vi "FGV_tristate_indicator_OBJ_test.vi"(6 "boolean_indicator_refnum":refnum<vi>, 7 "options":T1, 8 "error_in":errorcluster) -> (0 "error_out":errorcluster)   [LabVIEW 2019]
uses:
  FGV_tristate_indicator_OBJ_test.ctl
  _misc/AULocalize/SubVIs/Get Localized Phrase Compact Interface 1D.vi
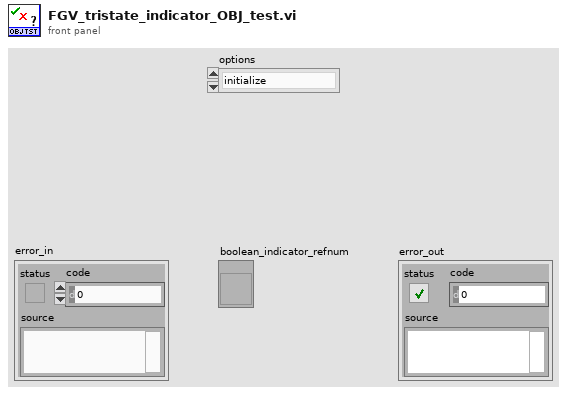
[diagram p1: front panel]
types:
  T1 = typedef "FGV_tristate_indicator_OBJ_test.ctl" = enum16{"initialize", "ready", "pending", "OK", "NOK", "part_NOK", "routing_NOK", "repeat_NOK", "timeout", "translate", "error"}
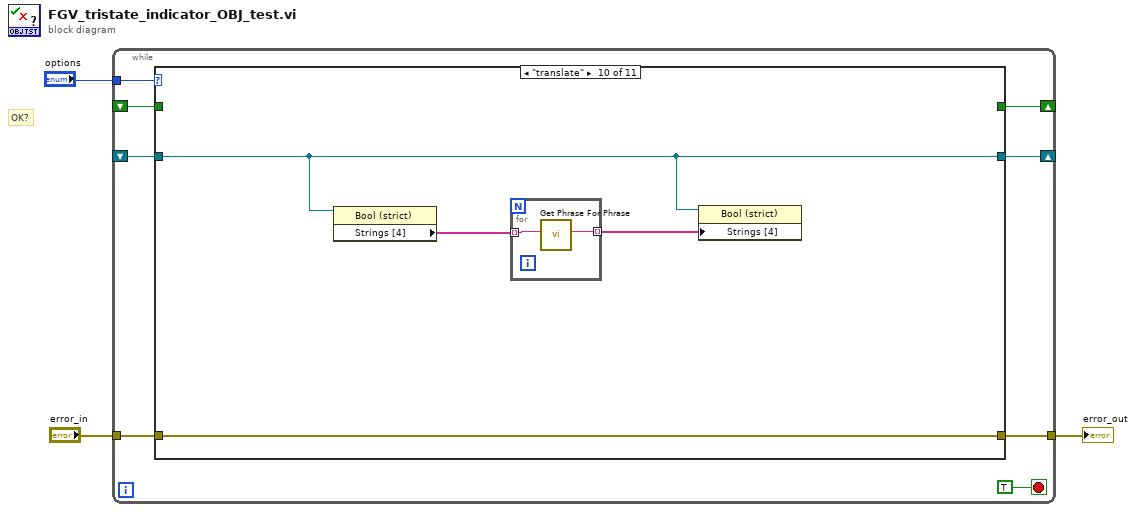
[diagram p0: block diagram]
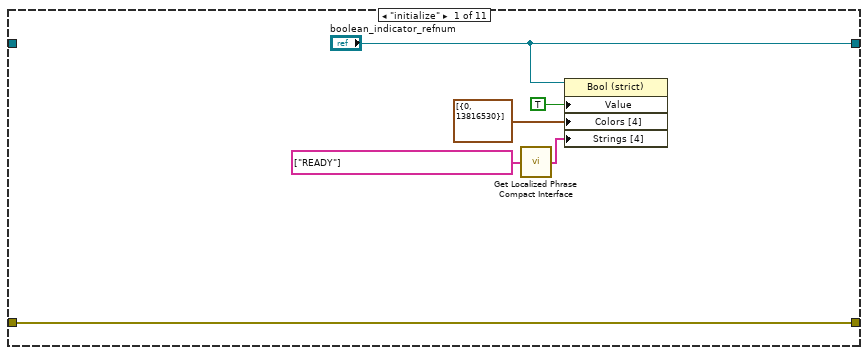
[diagram p2: hidden frame]
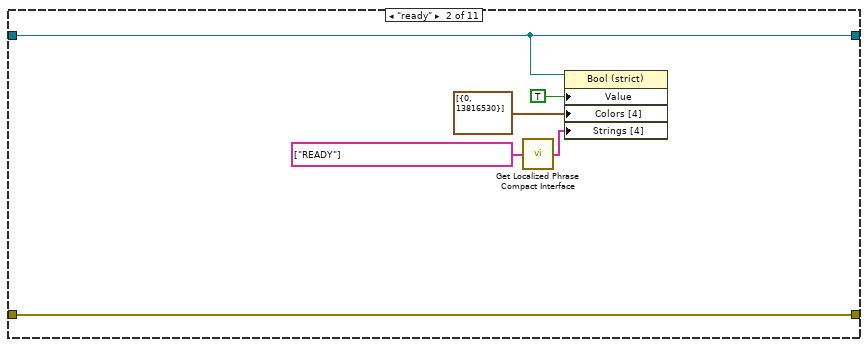
[diagram p3: hidden frame]
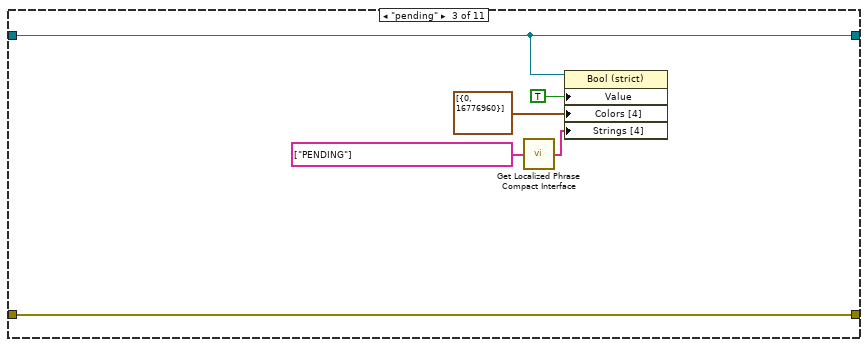
[diagram p4: hidden frame]
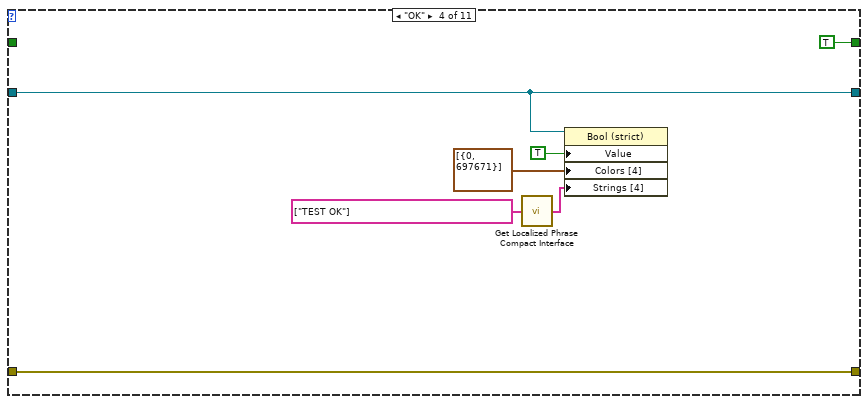
[diagram p5: hidden frame]
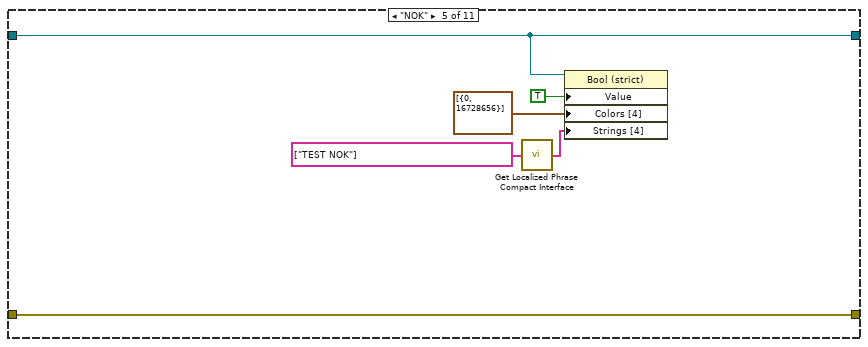
[diagram p6: hidden frame]
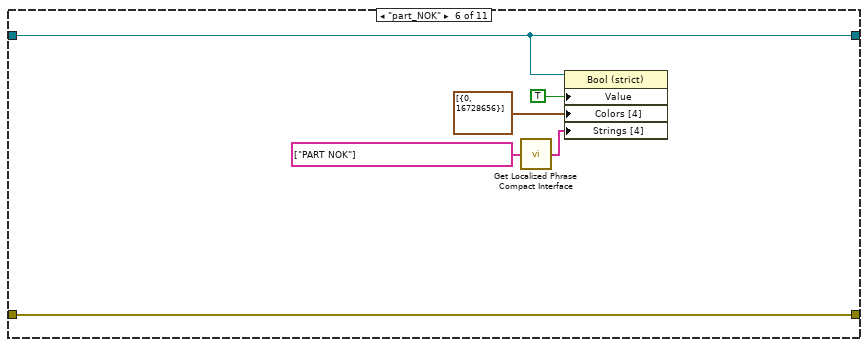
[diagram p7: hidden frame]
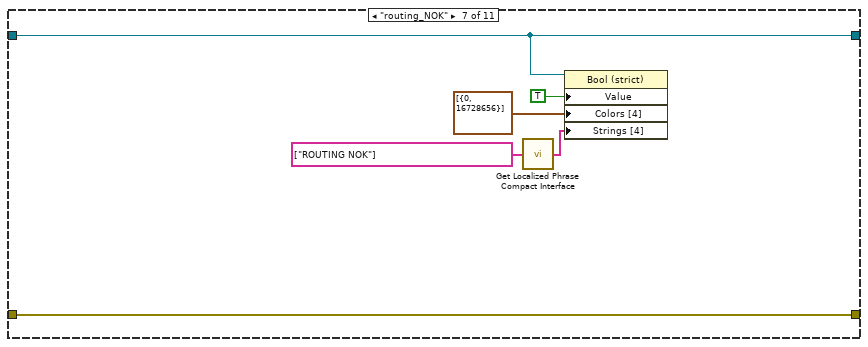
[diagram p8: hidden frame]
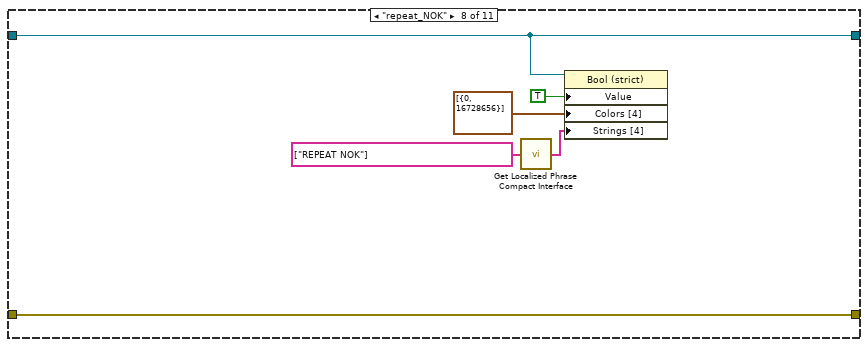
[diagram p9: hidden frame]
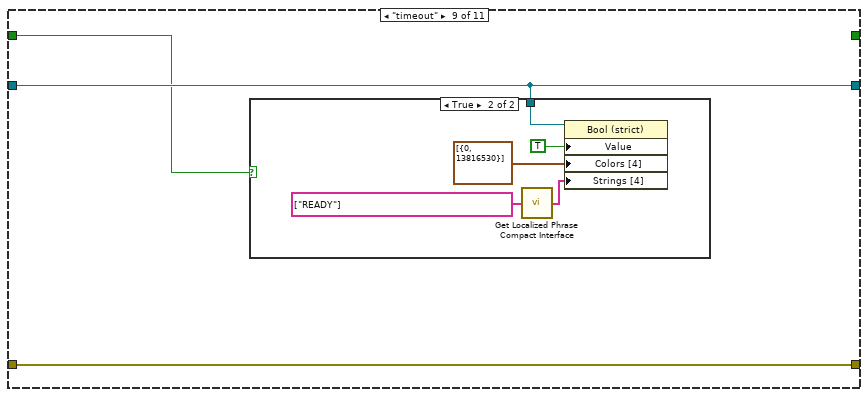
[diagram p10: hidden frame]
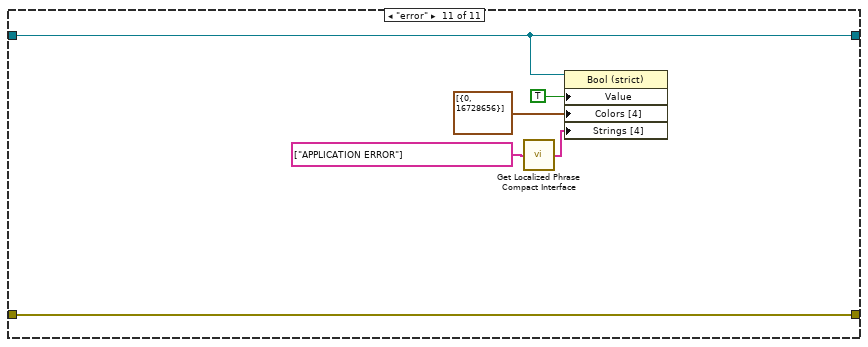
[diagram p12: hidden frame]
diagram:
  # "OK?"
  n1 = while {
    tunnel: "options" -> [w10]
    tunnel: [w9] -> w3
    tunnel: "error_in" -> [w8]
    shift-right: [w7] -> _
    shift-left: _ -> [w6]
    shift-right: [w5] -> _
    shift-left: _ -> [w4]
    stop <- TRUE stop-if-true
    n2 = case shown="\"translate\"" w10 {
      tunnel: [w17 w23 w29 w36 w42 w48 w54 w60 w63 w72 w80] -> w9
      tunnel: w8 -> [w17 w23 w29 w36 w42 w48 w54 w60 w63 w72 w80]
      tunnel: ["boolean_indicator_refnum" w20 w27 w33 w39 w45 w51 w57 w62 w71 w77] -> w7
      tunnel: w6 -> [_ w20 w27 w33 w39 w45 w51 w57 w62 w71 w77]
      tunnel: [_ _ _ TRUE _ _ _ _ _ _ _] -> w5
      tunnel: w4 -> [_ _ _ _ _ _ _ _ w61 _ _]
      frame "initialize" {
        n3 = call-poly "Get Localized Phrase Compact Interface.vi"("Key"=string[] ["READY"] ("Strings [4]")) -> ("Translated Phrase"=w12:string[])
        n4 = property on="Property Node" class="Bool (strict)"(reference="boolean_indicator_refnum", "Value"=TRUE ("Boolean"), "Colors [4]"=cluster{u32, u32}[] [{0, 13816530}], "Strings [4]"=w12) -> ()  [unwired: 1 in, 2 out]
      }
      frame "ready" {
        n5 = call-poly "Get Localized Phrase Compact Interface.vi"("Key"=string[] ["READY"] ("Strings [4]")) -> ("Translated Phrase"=w18:string[])
        n6 = property on="Property Node" class="Bool (strict)"(reference=w20, "Value"=TRUE ("Boolean"), "Colors [4]"=cluster{u32, u32}[] [{0, 13816530}], "Strings [4]"=w18) -> ()  [unwired: 1 in, 2 out]
      }
      frame "pending" {
        n7 = call-poly "Get Localized Phrase Compact Interface.vi"("Key"=string[] ["PENDING"] ("Strings [4]")) -> ("Translated Phrase"=w24:string[])
        n8 = property on="Property Node" class="Bool (strict)"(reference=w27, "Value"=TRUE ("Boolean"), "Colors [4]"=cluster{u32, u32}[] [{0, 16776960}], "Strings [4]"=w24) -> ()  [unwired: 1 in, 2 out]
      }
      frame "OK" {
        n9 = call-poly "Get Localized Phrase Compact Interface.vi"("Key"=string[] ["TEST OK"] ("Strings [4]")) -> ("Translated Phrase"=w31:string[])
        n10 = property on="Property Node" class="Bool (strict)"(reference=w33, "Value"=TRUE ("Boolean"), "Colors [4]"=cluster{u32, u32}[] [{0, 697671}], "Strings [4]"=w31) -> ()  [unwired: 1 in, 2 out]
      }
      frame "NOK" {
        n11 = call-poly "Get Localized Phrase Compact Interface.vi"("Key"=string[] ["TEST NOK"] ("Strings [4]")) -> ("Translated Phrase"=w38:string[])
        n12 = property on="Property Node" class="Bool (strict)"(reference=w39, "Value"=TRUE ("Boolean"), "Colors [4]"=cluster{u32, u32}[] [{0, 16728656}], "Strings [4]"=w38) -> ()  [unwired: 1 in, 2 out]
      }
      frame "part_NOK" {
        n13 = call-poly "Get Localized Phrase Compact Interface.vi"("Key"=string[] ["PART NOK"] ("Strings [4]")) -> ("Translated Phrase"=w43:string[])
        n14 = property on="Property Node" class="Bool (strict)"(reference=w45, "Value"=TRUE ("Boolean"), "Colors [4]"=cluster{u32, u32}[] [{0, 16728656}], "Strings [4]"=w43) -> ()  [unwired: 1 in, 2 out]
      }
      frame "routing_NOK" {
        n15 = call-poly "Get Localized Phrase Compact Interface.vi"("Key"=string[] ["ROUTING NOK"] ("Strings [4]")) -> ("Translated Phrase"=w49:string[])
        n16 = property on="Property Node" class="Bool (strict)"(reference=w51, "Value"=TRUE ("Boolean"), "Colors [4]"=cluster{u32, u32}[] [{0, 16728656}], "Strings [4]"=w49) -> ()  [unwired: 1 in, 2 out]
      }
      frame "repeat_NOK" {
        n17 = call-poly "Get Localized Phrase Compact Interface.vi"("Key"=string[] ["REPEAT NOK"] ("Strings [4]")) -> ("Translated Phrase"=w56:string[])
        n18 = property on="Property Node" class="Bool (strict)"(reference=w57, "Value"=TRUE ("Boolean"), "Colors [4]"=cluster{u32, u32}[] [{0, 16728656}], "Strings [4]"=w56) -> ()  [unwired: 1 in, 2 out]
      }
      frame "timeout" {
        n19 = case shown="True" w61 {
          tunnel: w62 -> [_ w66]
          frame False {
          }
          frame True {
            n20 = call-poly "Get Localized Phrase Compact Interface.vi"("Key"=string[] ["READY"] ("Strings [4]")) -> ("Translated Phrase"=w65:string[])
            n21 = property on="Property Node" class="Bool (strict)"(reference=w66, "Value"=TRUE ("Boolean"), "Colors [4]"=cluster{u32, u32}[] [{0, 13816530}], "Strings [4]"=w65) -> ()  [unwired: 1 in, 2 out]
          }
        }
      }
      frame "translate" {
        n22 = property on="Property Node" class="Bool (strict)"(reference=w71) -> ("Strings [4]"=w70:string[])  [unwired: 1 in, 2 out]
        n23 = for {
          tunnel: w70 -> [w74] mode=indexing
          tunnel: [w73] -> w69 mode=indexing
          n24 = call "Get Phrase For Phrase.vi"("Phrase"=w74) -> ("Phrase"=w73:string)  [unwired: 9 in, 1 out]
        }
        n25 = property on="Property Node" class="Bool (strict)"(reference=w71, "Strings [4]"=w69) -> ()  [unwired: 1 in, 2 out]
      }
      frame "error" {
        n26 = call-poly "Get Localized Phrase Compact Interface.vi"("Key"=string[] ["APPLICATION ERROR"] ("Strings [4]")) -> ("Translated Phrase"=w75:string[])
        n27 = property on="Property Node" class="Bool (strict)"(reference=w77, "Value"=TRUE ("Boolean"), "Colors [4]"=cluster{u32, u32}[] [{0, 16728656}], "Strings [4]"=w75) -> ()  [unwired: 1 in, 2 out]
      }
    }
  }
  "error_out" <- w3
